vi "EHL Timeout EHLC.vi"(8 "error in":errorcluster, 10 "This VI":refnum<vi>, 11 "Message Log in":refnum<class "Message Log.lvclass">) -> (0 "error out":errorcluster, 2 "# elements in queue":i32, 3 "Message Log out":refnum<class "Message Log.lvclass">)   [LabVIEW 2017, in "Message Log.lvclass"]
uses:
  Message Log.lvclass
  C:/Program Files (x86)/National Instruments/LabVIEW 2017/vi.lib/addons/_Workers/Library/Classes/Worker/Worker.lvclass
  <vilib>/addons/_Workers/Library/Classes/Worker/Worker.lvclass/Worker.ctl
  <vilib>/addons/_Workers/Library/Classes/Message Queue/Message Queue.lvclass/Message Queue.ctl
  Message Log.lvclass/Message Log.ctl
  <vilib>/addons/_Workers/Library/Classes/Worker/Worker.lvclass
  <vilib>/addons/_Workers/Library/Classes/Message Queue/Message Queue.lvclass
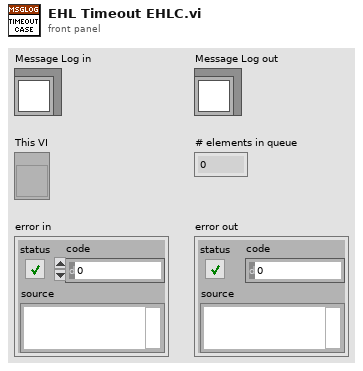
[diagram p1: front panel]
types:
  T1 = typedef "Workers.lvlib/Message Queue.lvclass/DVR Contents.ctl" = cluster{"# Waiting":u32, "Buffers":refnum<queue>[], "Wait Msg":refnum<queue>, "Wait Prior":refnum<queue>}
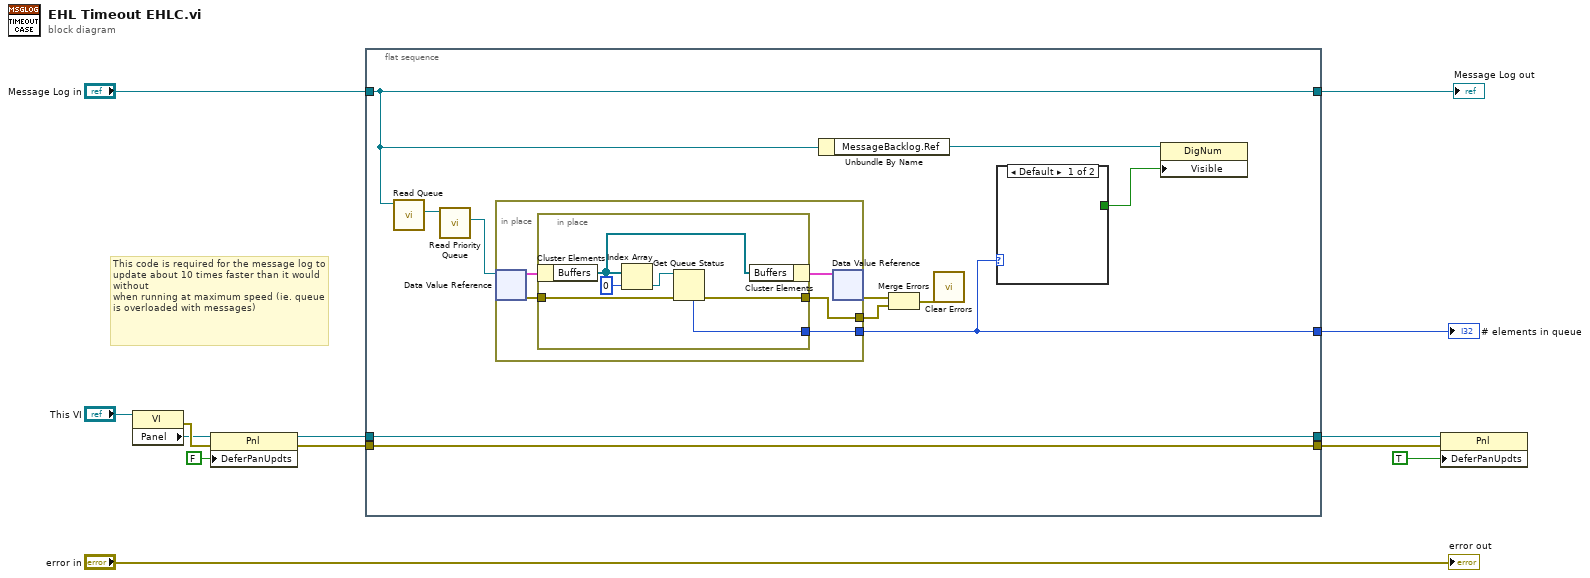
[diagram p0: block diagram]
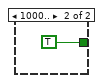
[diagram p2: hidden frame]
diagram:
  # "This code is required for the message log to update about 10 times faster than it would without\nwhen running at maximum speed (ie. queue is overloaded with messages)"
  n1 = property class="VI"(reference="This VI") -> (error out=w12:errorcluster, "Panel"=w9:refnum<vi>)  [unwired: 1 in, 1 out]
  n2 = property class="Pnl"(reference=w9, error in=w12, "DeferPanUpdts"=FALSE ("Defer Panel Updates")) -> (reference out=w4:refnum<vi>, error out=w5:errorcluster)
  n3 = flat-sequence {
    tunnel: [w14] -> w13
    tunnel: "Message Log in" -> [w15]
    tunnel: [w17] -> w6
    tunnel: w5 -> [w17]
    tunnel: w4 -> [w16]
    tunnel: [w16] -> w3
    tunnel: [w15] -> w1
    frame #0 {
      n4 = call <vilib>:"Read Queue.vi"("Worker_"=w15) -> ("Message Queue out"=w22:refnum<class "Message Queue.lvclass">)  [unwired: 9 in, 1 out]
      n5 = call <vilib>:"Read Priority Queue.vi"("Message Queue"=w22) -> ("Priority Queue"=w23:refnum<data-value>)  [unwired: 9 in, 1 out]
      n6 = in-place {
        in-place-border: [w26] -> w21
        in-place-border: [w28] -> w14
        n7 = in-place-dvr #1(w23) -> (w30:T1, w27:errorcluster)
        n8 = in-place {
          in-place-border: [w32] -> w28
          in-place-border: w27 -> [w33]
          in-place-border: [w34] -> w26
          n9 = in-place-cluster #2(w30) -> ("Buffers"=w36:refnum<queue>[])
          n10 = Index Array(array=w36, index=0) -> (element=w35:refnum<queue>)
          n11 = Get Queue Status(queue=w35, error in (no error)=w33) -> (error out=w34:errorcluster, # elements in queue=w32:i32)  [unwired: 1 in, 6 out]
          n12 = in-place-cluster #2("Buffers"=w36) -> (w29:T1)
        }
        n13 = in-place-dvr #1(w29) -> (w20:errorcluster)  [unwired: 1 out]
      }
      n14 = Unbundle By Name(w15) -> ("MessageBacklog.Ref"=w19:refnum<vi>)
      n15 = Merge Errors(w20, w21) -> (w24:errorcluster)
      n16 = call <vilib>:"Clear Errors.vi"("error in (no error)"=w24) -> ()  [unwired: 5 in, 2 out]
      n17 = case shown="Default" w14 {
        tunnel: [_ TRUE ("Blinking")] -> w18
        frame Default {
        }
        frame 1000.. {
        }
      }
      n18 = property class="DigNum"(reference=w19, "Visible"=w18) -> ()  [unwired: 1 in, 2 out]
    }
  }
  n19 = property class="Pnl"(reference=w3, error in=w6, "DeferPanUpdts"=TRUE ("Defer Panel Updates")) -> ()  [unwired: 2 out]
  "Message Log out" <- w1
  "error out" <- "error in"
  "# elements in queue" <- w13
